vi "Save Recall Setup Data.vi"(8 "error in (no error)":errorcluster, 9 "Memory Location (1)":i32=1, 10 "Operation (0: Save)":i32(ring) items=["Save", "Recall"], 11 "VISA resource name":refnum<visa-resource-name>) -> (0 "error out":errorcluster, 3 "VISA resource name out":refnum<visa-resource-name>)   [LabVIEW 2020, in "Keithley 2600 Series.lvlib"]
doc: "Saves or recalls the instrument setting."
uses:
  <instrlib>/Keithley 2600 Series/Keithley 2600 Series.lvlib
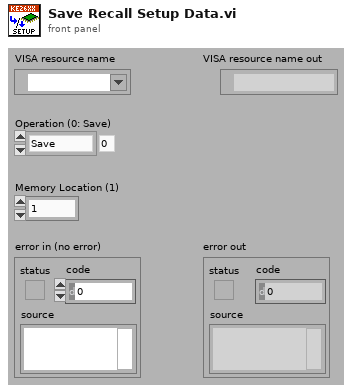
[diagram p1: front panel]
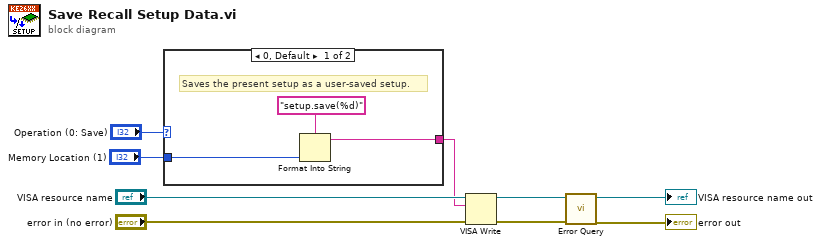
[diagram p0: block diagram]
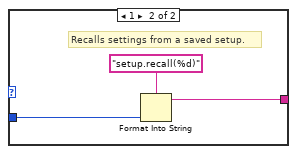
[diagram p2: hidden frame]
diagram:
  n1 = case shown="0, Default" "Operation (0: Save)" {
    tunnel: "Memory Location (1)" -> [w11 w14]
    tunnel: [w10 w13] -> w1
    frame 0, Default {
      # "Saves the present setup as a user-saved setup."
      n2 = Format Into String(format string="setup.save(%d)", w11) -> (resulting string=w10:string)  [unwired: 2 in, 1 out]
    }
    frame 1 {
      # "Recalls settings from a saved setup."
      n3 = Format Into String(format string="setup.recall(%d)", w14) -> (resulting string=w13:string)  [unwired: 2 in, 1 out]
    }
  }
  n4 = VISA Write(VISA resource name="VISA resource name", write buffer=w1, error in (no error)="error in (no error)") -> (VISA resource name out=w7:refnum<visa-resource-name>, error out=w6:errorcluster)  [unwired: 1 out]
  n5 = call <instrlib>:"Error Query.vi"("error in (no error)"=w6, "VISA resource name"=w7) -> ("error out"=→"error out":errorcluster, "VISA resource name out"=→"VISA resource name out":refnum<visa-resource-name>)  [unwired: 6 in, 2 out]
